vi "signal data analysis.vi"() -> ()   [LabVIEW 2012]
panel:
  in  "Filename":path=path "C:/Users/Vedant Bhoj/Documents/Vedant labview/DAY 4/signal data.lvm"
  out "Signals":dynamicdata(graph)
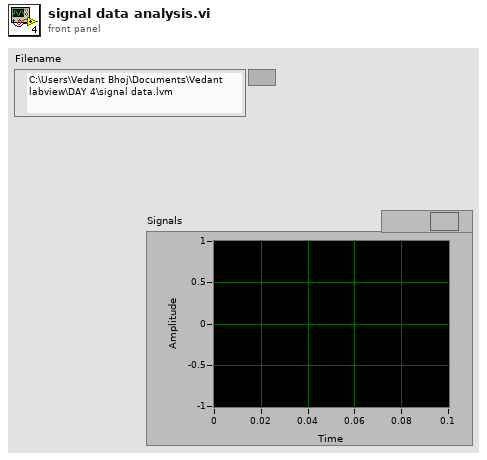
[diagram p1: front panel]
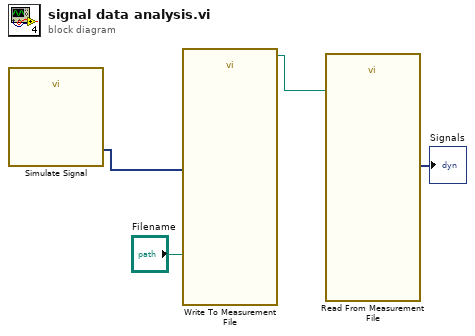
[diagram p0: block diagram]
diagram:
  n1 = call "Simulate Signal"() -> ("Sine"=w3:dynamicdata)  [unwired: 14 in, 1 out]
  n2 = call "Write To Measurement File"("Signals"=w3, "Filename"="Filename") -> ("Filename Out"=w4:path)  [unwired: 15 in, 2 out]
  n3 = call "Read From Measurement File"("Filename"=w4) -> ("Signals"=→"Signals":dynamicdata)  [unwired: 5 in, 5 out]
